vi "calcControllerOutput.vi"(8 "error in (no error)":errorcluster, 9 "loopPeriod":dbl[unit]=5000.0 min=10.0 max=5000.0, 10 "step rate limit (mag)":dbl[unit]=5000000.0 min=10000.0 max=5000000.0, 11 "SystemController in":refnum<class "SystemController.lvclass">) -> (0 "error out":errorcluster, 2 "Compensator Output":T1={"Compression Pressure Transducer Setpoint"=5000.0, "Tension Pressure Transducer Setpoint"=5000.0, "Flow Control Valve Setpoint"=5000.0} {"Flow Control Valve Setpoint" min=10.0 max=5000.0; "Tension Pressure Transducer Setpoint" min=10.0 max=5000.0; "Compression Pressure Transducer Setpoint" min=10.0 max=5000.0}, 3 "SystemController out":refnum<class "SystemController.lvclass">)   [LabVIEW 2013, in "SystemController.lvclass"]
uses:
  SystemController.lvclass
  Typedefs/CompensatorOutput.ctl
  SystemController.lvclass/SystemController.ctl
  DualActingPneumaticCylinder/DualActingPneumaticCylinder.lvclass/DualActingPneumaticCylinder.ctl
  DualActingPneumaticCylinder/DualActingPneumaticCylinder.lvclass
  PressureTransducerCompensator/PressureTransducerCompensator.lvclass
  FlowControlValveCompensator/FlowControlValveCompensator.lvclass
  Typedefs/FAMTTypedefs.lvlib
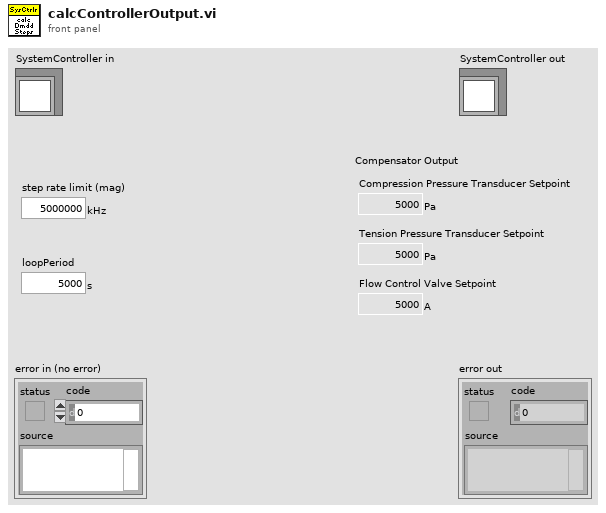
[diagram p1: front panel]
types:
  T1 = typedef "FAMTTypedefs.lvlib/CompensatorOutput.ctl" = cluster{"Compression Pressure Transducer Setpoint":dbl[unit], "Tension Pressure Transducer Setpoint":dbl[unit], "Flow Control Valve Setpoint":dbl[unit]}
  T2 = typedef "FAMTTypedefs.lvlib/ForceSetpoint.ctl" = dbl[unit]
  T3 = typedef "FAMTTypedefs.lvlib/PressureTransducerSetpoint.ctl" = cluster{"Compression":dbl[unit], "Tension":dbl[unit]}
  T4 = typedef "FAMTTypedefs.lvlib/FlowControlValveSetpoint.ctl" = dbl[unit]
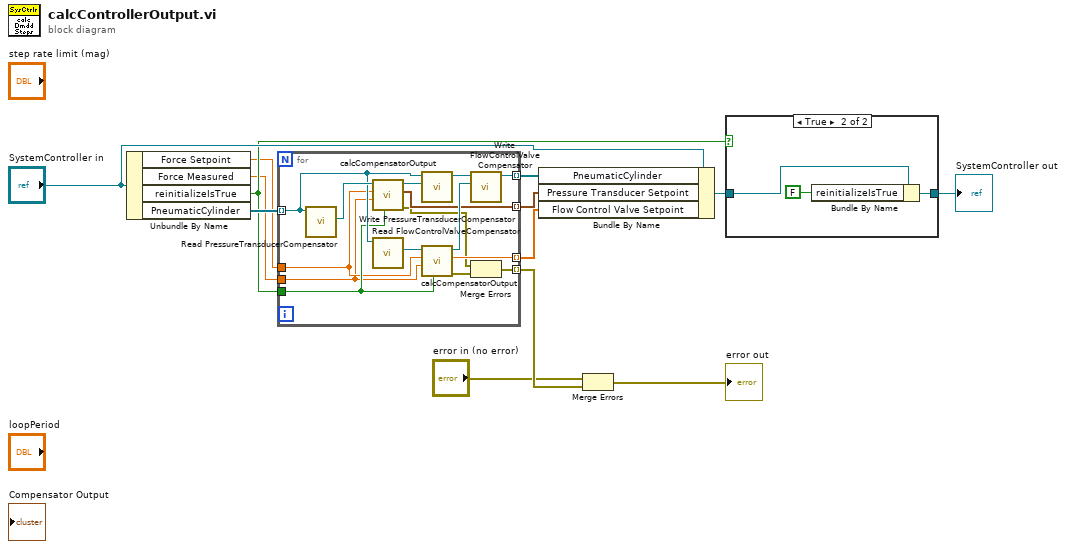
[diagram p0: block diagram]
diagram:
  n1 = Unbundle By Name("SystemController in") -> ("Force Setpoint"=w5:T2, "Force Measured"=w4:T2, "reinitializeIsTrue"=w6:bool, "PneumaticCylinder"=w12:refnum<class "DualActingPneumaticCylinder.lvclass">[])
  n2 = for {
    tunnel: w12 -> [w25] mode=indexing
    tunnel: [w22] -> w10 mode=indexing
    tunnel: [w21] -> w8 mode=indexing
    tunnel: [w20] -> w7 mode=indexing
    tunnel: w6 -> [w19]
    tunnel: w5 -> [w18]
    tunnel: w4 -> [w17]
    tunnel: [w14] -> w3 mode=indexing
    n3 = call "Read PressureTransducerCompensator.vi"("DualActingPneumaticCylinder in"=w25) -> ("PressureTransducerCompensator.lvclass"=w28:refnum<class "PressureTransducerCompensator.lvclass">)  [unwired: 9 in, 1 out]
    n4 = call "calcCompensatorOutput.vi"("reinitializeIsTrue"=w19, "Force Measured"=w17, "Force Setpoint"=w18, "PressureTransducerCompensator in"=w28) -> ("error out"=w16:errorcluster, "Pressure Transducer Setpoint"=w21:T3, "PressureTransducerCompensator out"=w27:refnum<class "PressureTransducerCompensator.lvclass">)  [unwired: 5 in]
    n5 = call "Read FlowControlValveCompensator.vi"("DualActingPneumaticCylinder in"=w25) -> ("FlowControlValveCompensator.lvclass"=w26:refnum<class "FlowControlValveCompensator.lvclass">)  [unwired: 9 in, 1 out]
    n6 = call "Write PressureTransducerCompensator.vi"("PressureTransducerCompensator.lvclass"=w27, "DualActingPneumaticCylinder in"=w25) -> ("DualActingPneumaticCylinder out"=w23:refnum<class "DualActingPneumaticCylinder.lvclass">)  [unwired: 9 in]
    n7 = call "calcCompensatorOutput.vi"("reinitializeIsTrue"=w19, "Force Measured"=w17, "Force Setpoint"=w18, "FlowControlValveCompensator in"=w26) -> ("error out"=w15:errorcluster, "Flow Control Valve Setpoint"=w20:T4, "FlowControlValveCompensator out"=w24:refnum<class "FlowControlValveCompensator.lvclass">)  [unwired: 5 in]
    n8 = call "Write FlowControlValveCompensator.vi"("FlowControlValveCompensator.lvclass"=w24, "DualActingPneumaticCylinder in"=w23) -> ("DualActingPneumaticCylinder out"=w22:refnum<class "DualActingPneumaticCylinder.lvclass">)  [unwired: 9 in]
    n9 = Merge Errors(w16, w15) -> (w14:errorcluster)
  }
  n10 = Bundle By Name(cluster="SystemController in", "PneumaticCylinder"=w10, "Pressure Transducer Setpoint"=w8, "Flow Control Valve Setpoint"=w7) -> (w9:refnum<class "SystemController.lvclass">)
  n11 = Merge Errors("error in (no error)", w3) -> (→"error out":errorcluster)
  n12 = case shown="True" w6 {
    tunnel: [w29 w31] -> w13
    tunnel: w9 -> [w29 w32]
    frame False {
    }
    frame True {
      n13 = Bundle By Name(cluster=w32, "reinitializeIsTrue"=FALSE ("reinitialize? (F)")) -> (w31:refnum<class "SystemController.lvclass">)
    }
  }
  "SystemController out" <- w13
